vi "Read RefreshTime.vi"(8 "error in (no error)":errorcluster, 11 "AcPwrBase in":refnum<class "AcPwrBase.lvclass">) -> (0 "error out":errorcluster, 2 "RefreshTime":dbl, 3 "AcPwrBase out":refnum<class "AcPwrBase.lvclass">)   [LabVIEW 2014, in "AcPwrPlugins.lvlib" / "AcPwrBase.lvclass"]
uses:
  AcPwrBase.lvclass
  AcPwrBase.lvclass/AcPwrBase.ctl
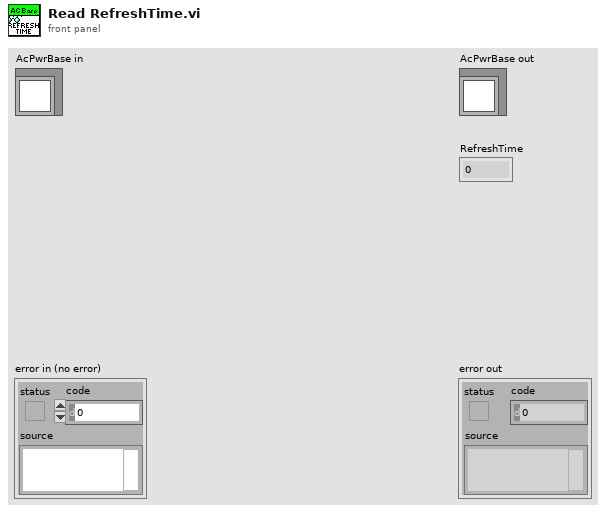
[diagram p1: front panel]
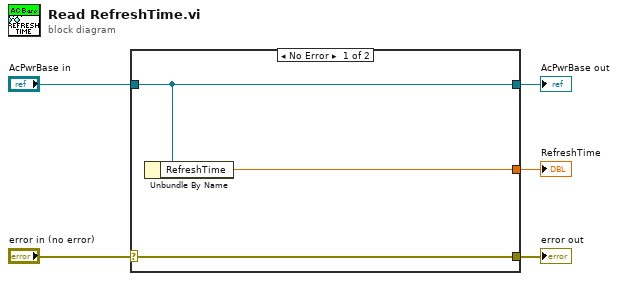
[diagram p0: block diagram]
diagram:
  n1 = case shown="No Error" "error in (no error)" {
    selector: "error in (no error)" -> [w8 w9]
    tunnel: [w8 w9] -> w4
    tunnel: [w7 w10] -> w2
    tunnel: "AcPwrBase in" -> [w7 w10]
    tunnel: [w6 _] -> w1
    frame No Error {
      n2 = Unbundle By Name(w7) -> ("RefreshTime"=w6:dbl)
    }
    frame Error {
    }
  }
  "error out" <- w4
  "AcPwrBase out" <- w2
  "RefreshTime" <- w1
